vi "uActor_PreInit.vi"(8 "error in (no error)":errorcluster, 11 "uObserver in":refnum<class "uObserver.lvclass">) -> (0 "error out":errorcluster, 3 "uObserver out":refnum<class "uObserver.lvclass">)   [LabVIEW 2021, in "uFramework_pack_uActor.lvlib" / "uObserver.lvclass"]
uses:
  uObserver.lvclass
  uObserver.lvclass/uObserver.ctl
  Bin/uFramework.lvlibp/uActor/uActor.lvclass
  U:/Projects/uFramework/Bin/uFramework.lvlibp/uActor/uActor.lvclass
  U:/Projects/uFramework/Bin/uFramework.lvlibp/uTransport/uTransport.lvclass
  U:/Projects/uFramework/Src/uFramework_pack_uActor/uObserver/uObserver.lvclass
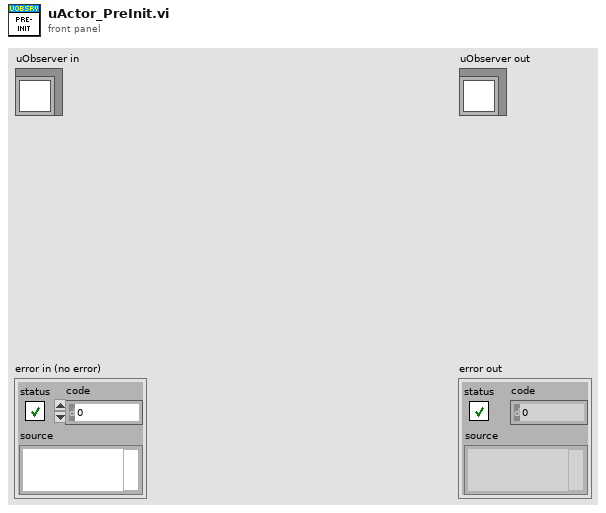
[diagram p1: front panel]
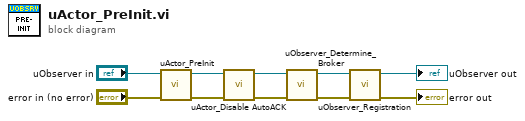
[diagram p0: block diagram]
diagram:
  n1 = call-parent "uActor_PreInit.vi"("error in (no error)"="error in (no error)", "uActor in"="uObserver in") -> ("error out"=w4:errorcluster, "uActor out"=w1:refnum<class "uObserver.lvclass">)  [unwired: 8 in]
  n2 = call "uActor_Disable AutoACK.vi"("error in (no error)"=w4, "uActor in"=w1) -> ("error out"=w6:errorcluster, "uActor out"=w5:refnum<class "uObserver.lvclass">)  [unwired: 8 in]
  n3 = call-dynamic "uObserver_Determine_Broker.vi"("error in (no error)"=w6, "uObserver in"=w5) -> ("error out"=w8:errorcluster, "uObserver out"=w7:refnum<class "uObserver.lvclass">)  [unwired: 8 in]
  n4 = call-dynamic "uObserver_Registration.vi"("error in (no error)"=w8, "uObserver in"=w7) -> ("error out"=→"error out":errorcluster, "uObserver out"=→"uObserver out":refnum<class "uObserver.lvclass">)  [unwired: 8 in]
